vi "tb_BRAM Control Logic.vi"() -> ()   [LabVIEW 2011]
uses:
  <instrlib>/FlexRIO/Libraries/Helper VIs/NI FlexRIO Helper VIs.lvlib
panel:
  out "Write COunts":u16[](array[numeric])=[0, 1, 2, 3, 4, 5, 6, 7, 8, 9, 10, 11, 12, 13, 14, 15, 16, 17, 18, 19, 20, 21, 22, 23, 24, 25, 26, 27, 28, 29, 30, 31, 32, 33, 34, 35, 36, 37, 38, 39, 40, 41, 42, 43, 44, 45, 46, 47, 48, 49, 50, 51, 52, 53, 54, 55, 56, 57, 58, 59, 60, 61, 62, 63, 64, 65, 66, 67, 68, 69, 70, 71, 72, 73, 74, 75, 76, 77, 78, 79, 80, 81, 82, 83, 84, 85, 86, 87, 88, 89, 90, 91, 92, 93, 94, 95, 96, 97, 98, 99]
  out "Iterations":i32=99
  out "Blocks Read":fxp<+,3,3>[](array[numeric])
  out "Blocks Written":fxp<+,3,3>[](array[numeric])
  out "Write Count End?":bool[](array[boolean])
  in  "Iterations":i32=100
  out "Read Valid":bool[](array[boolean])
  out "Bank0 Write":bool[](array[boolean])
  out "Read Address":u16[](array[numeric])
  in  "Read Count":u16=2
  in  "Write Count":u16=4
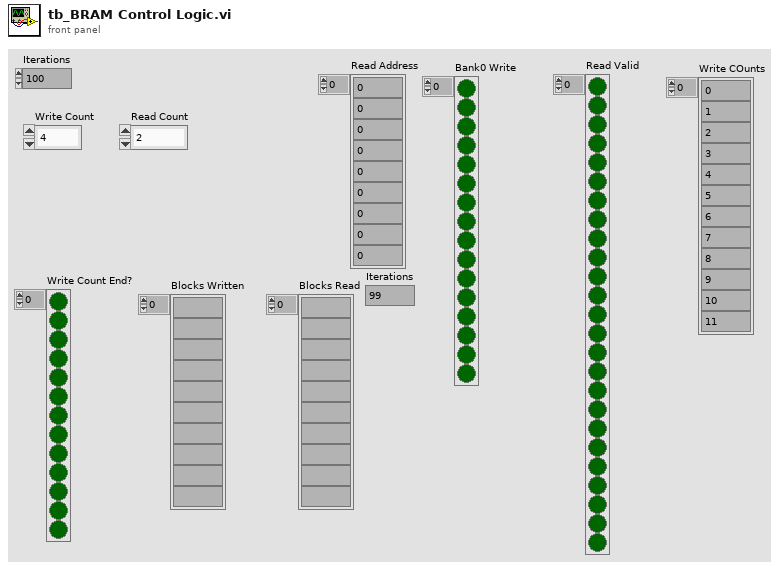
[diagram p1: front panel]
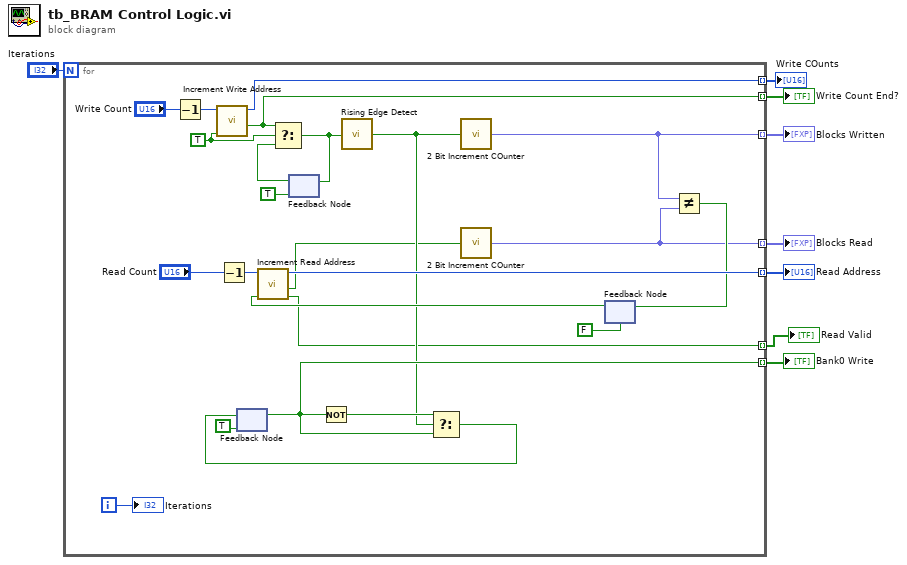
[diagram p0: block diagram]
diagram:
  n1 = for {
    N: "Iterations" -> [_]
    tunnel: [w29] -> w8 mode=indexing
    tunnel: [w28] -> w7 mode=indexing
    tunnel: [w16] -> w5 mode=indexing
    tunnel: [w15] -> w4 mode=indexing
    tunnel: [w14] -> w3 mode=indexing
    tunnel: [w10] -> w2 mode=indexing
    tunnel: [w9] -> w1 mode=indexing
    i -> [w12]
    w30 = TRUE ("Input Valid")
    n2 = Decrement(x="Write Count") -> (x-1=w25:u16)
    n3 = call <userlib>:"Increment Write Address.vi"("INC?"=w30, "rollover"=w25) -> ("roll over"=w16:bool, "count"=w10:u16)  [unwired: 7 in, 1 out]
    n4 = Decrement(x="Read Count") -> (x-1=w26:u16)
    n5 = feedback #1(TRUE) -> (w28:bool)
    n6 = feedback #2(TRUE ("roll over")) -> (w19:bool)
    n7 = Select(t=w16, s=w30, f=w19) -> (s? t:f=w20:bool)
    n8 = feedback-in #2(w20) -> ()
    n9 = Not(x=w28) -> (.not. x?=w18:bool)
    n10 = call <instrlib>:"Rising Edge Detect.vi"("signal"=w20) -> ("edge detected"=w13:bool)  [unwired: 14 in]
    n11 = Select(t=w18, s=w13, f=w28) -> (s? t:f=w22:bool)
    n12 = feedback-in #1(w22) -> ()
    n13 = call <userlib>:"2 Bit Increment COunter.vi"("Increment"=w13) -> ("Counter Value"=w15:fxp<+,3,3>)  [unwired: 14 in]
    n14 = feedback #3(FALSE) -> (w24:bool)
    n15 = call <userlib>:"Increment Read Address.vi"("INC?"=w24, "rollover"=w26) -> ("Output Valid"=w9:bool, "roll over"=w11:bool, "count"=w29:u16)  [unwired: 7 in]
    n16 = call <userlib>:"2 Bit Increment COunter.vi"("Increment"=w11) -> ("Counter Value"=w14:fxp<+,3,3>)  [unwired: 14 in]
    n17 = Not Equal?(x=w15, y=w14) -> (x != y?=w27:bool)
    n18 = feedback-in #3(w27) -> ()
    "Iterations" <- w12
  }
  "Read Address" <- w8
  "Bank0 Write" <- w7
  "Read Valid" <- w1
  "Write Count End?" <- w5
  "Blocks Written" <- w4
  "Blocks Read" <- w3
  "Write COunts" <- w2
